vi "실습 1-2 더하기빼기.vi"() -> ()   [LabVIEW 2014]
panel:
  out "A 4":dbl
  out "A 3":dbl
  in  "A 2":dbl
  in  "A":dbl
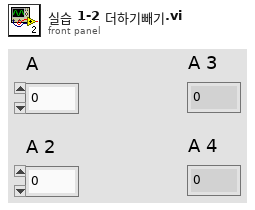
[diagram p1: front panel]
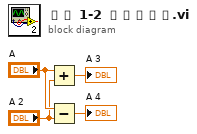
[diagram p0: block diagram]
diagram:
  n1 = Add(x="A", y="A 2") -> (x+y=→"A 3":dbl)
  n2 = Subtract(x="A", y="A 2") -> (x-y=→"A 4":dbl)
